vi "ChaseBoat.vi"(3 "Base Station data rec'd":string, 4 "inPriors":T1(array[cluster]), 5 "Tug letter":string="G") -> (0 "outPriors":T1(array[cluster]), 1 "predictedY":dbl, 2 "predictedX":dbl)   [LabVIEW 2012]
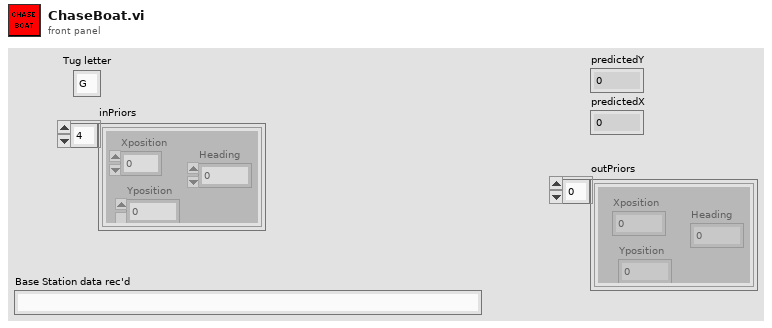
[diagram p1: front panel]
types:
  T1 = cluster{"Xposition":dbl, "Yposition":dbl, "Heading":dbl}[]
  T2 = cluster{"regular expression":string, i32, i32, i32}
  T3 = cluster{"Xposition":dbl, "Yposition":dbl, "Heading":dbl}
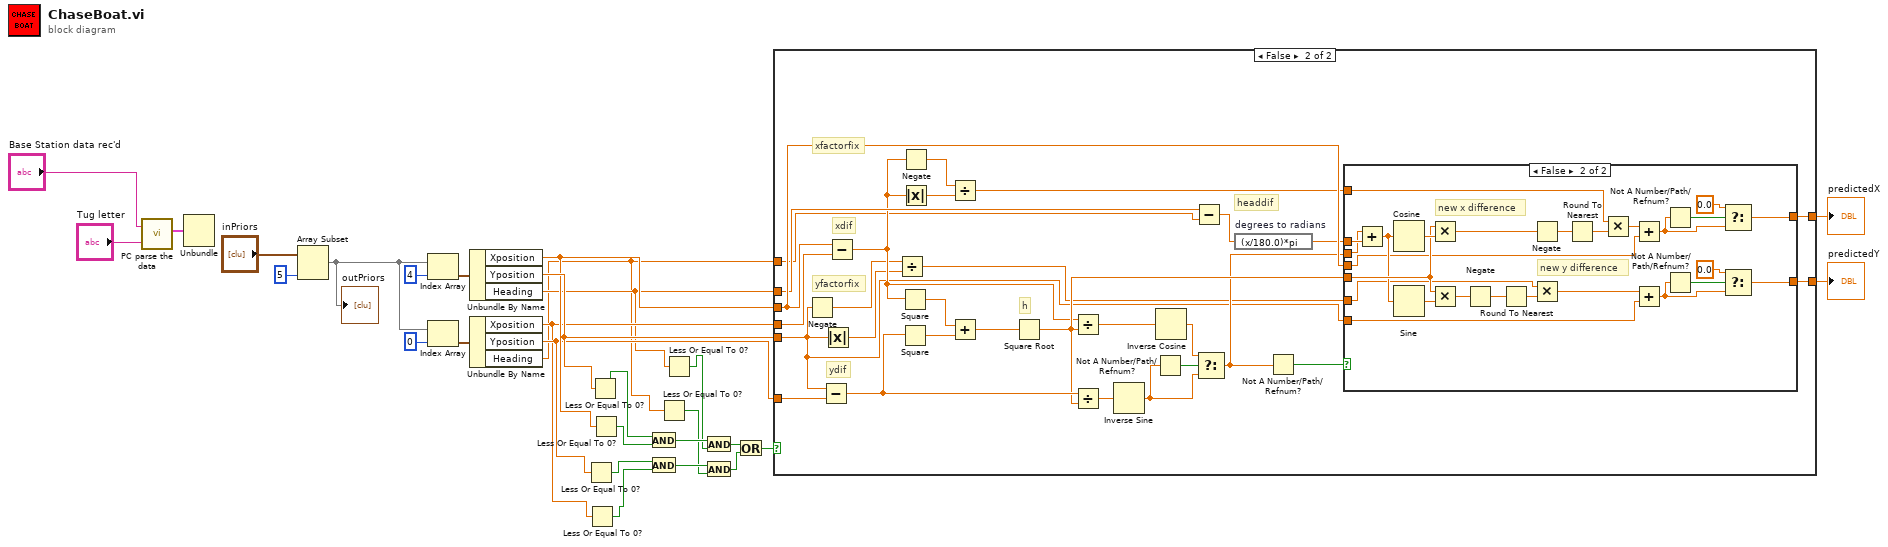
[diagram p0: block diagram]
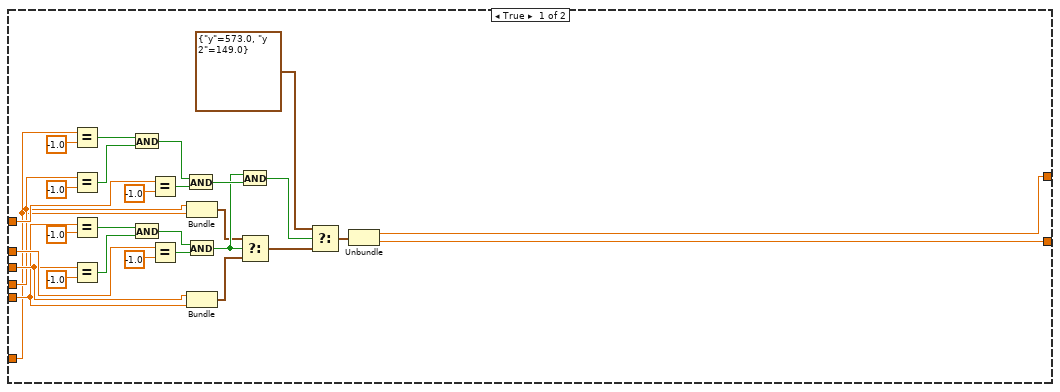
[diagram p2: hidden frame]
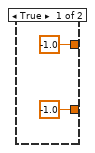
[diagram p3: hidden frame]
diagram:
  n1 = call "PC parse the data.vi"("Nav String"="Base Station data rec'd", "Tug"="Tug letter") -> ("Tug Location"=w27:T2)  [unwired: 3 out]
  n2 = Unbundle(w27) -> ()  [unwired: 4 out]
  n3 = Array Subset(array="inPriors", length=5) -> (w25:T1)  [unwired: 1 in]
  "outPriors" <- w25
  n4 = Index Array(array=w25, index=4) -> (element=w21:T3)
  n5 = Index Array(array=w25, index=0) -> (element=w22:T3)
  n6 = Unbundle By Name(w21) -> ("Xposition"=w9:dbl, "Yposition"=w12:dbl, "Heading"=w3:dbl)
  n7 = Unbundle By Name(w22) -> ("Xposition"=w5:dbl, "Yposition"=w7:dbl, "Heading"=w2:dbl)
  n8 = Less Or Equal To 0?(x=w7) -> (x <= 0?=w8:bool)
  n9 = Less Or Equal To 0?(x=w5) -> (x <= 0?=w6:bool)
  n10 = Less Or Equal To 0?(x=w12) -> (x <= 0?=w11:bool)
  n11 = Less Or Equal To 0?(x=w9) -> (x <= 0?=w10:bool)
  n12 = And(x=w11, y=w10) -> (x .and. y?=w17:bool)
  n13 = And(x=w8, y=w6) -> (x .and. y?=w16:bool)
  n14 = Less Or Equal To 0?(x=w2) -> (x <= 0?=w1:bool)
  n15 = Less Or Equal To 0?(x=w3) -> (x <= 0?=w4:bool)
  n16 = And(x=w17, y=w4) -> (x .and. y?=w14:bool)
  n17 = And(x=w16, y=w1) -> (x .and. y?=w15:bool)
  n18 = Or(x=w14, y=w15) -> (x .or. y?=w13:bool)
  n19 = case shown="False" w13 {
    tunnel: w5 -> [w36 w88]
    tunnel: w7 -> [w35 w87]
    tunnel: w9 -> [w39 w83]
    tunnel: [w30 w82] -> w19
    tunnel: [w31 w81] -> w18
    tunnel: w3 -> [w52 w70]
    tunnel: w12 -> [w38 w63]
    tunnel: w2 -> [w44 w60]
    frame True {
      n20 = Equal?(x=w35, y=-1.0) -> (x = y?=w50:bool)
      n21 = Equal?(x=w36, y=-1.0) -> (x = y?=w51:bool)
      n22 = Equal?(x=w38, y=-1.0) -> (x = y?=w58:bool)
      n23 = Equal?(x=w39, y=-1.0) -> (x = y?=w59:bool)
      n24 = And(x=w50, y=w51) -> (x .and. y?=w49:bool)
      n25 = And(x=w58, y=w59) -> (x .and. y?=w57:bool)
      n26 = Equal?(x=w44, y=-1.0) -> (x = y?=w48:bool)
      n27 = Equal?(x=w52, y=-1.0) -> (x = y?=w56:bool)
      n28 = And(x=w49, y=w48) -> (x .and. y?=w43:bool)
      n29 = Bundle("Xposition"=w36, "Yposition"=w35) -> (w34:cluster{"Xposition":dbl, "Yposition":dbl})  [unwired: 1 in]
      n30 = And(x=w57, y=w56) -> (x .and. y?=w40:bool)
      n31 = Bundle("Xposition"=w39, "Yposition"=w38) -> (w37:cluster{"Xposition":dbl, "Yposition":dbl})  [unwired: 1 in]
      n32 = And(x=w40, y=w43) -> (x .and. y?=w42:bool)
      n33 = Select(t=w34, s=w40, f=w37) -> (s? t:f=w33:cluster{"Xposition":dbl, "Yposition":dbl})
      n34 = Select(t=cluster{"y":dbl, "y 2":dbl} {"y"=573.0, "y 2"=149.0}, s=w42, f=w33) -> (s? t:f=w32:cluster{"Xposition":dbl, "Yposition":dbl})
      n35 = Unbundle(w32) -> ("Xposition"=w31:dbl, "Yposition"=w30:dbl)
    }
    frame False {
      # "yfactorfix"
      # "xfactorfix"
      # "h"
      # "xdif"
      # "ydif"
      # "headdif"
      n36 = Negate(x=w63) -> (-x=w65:dbl)
      n37 = Subtract(x=w63, y=w87) -> (x-y=w79:dbl)
      n38 = Absolute Value(x=w63) -> (abs(x)=w64:dbl)
      n39 = Subtract(x=w83, y=w88) -> (x-y=w68:dbl)
      n40 = Divide(x=w65, y=w64) -> (x/y=w62:dbl)
      n41 = Square(x=w68) -> (x^2=w86:dbl)
      n42 = Square(x=w79) -> (x^2=w85:dbl)
      n43 = Negate(x=w68) -> (-x=w67:dbl)
      n44 = Absolute Value(x=w68) -> (abs(x)=w66:dbl)
      n45 = Divide(x=w67, y=w66) -> (x/y=w61:dbl)
      n46 = Add(x=w86, y=w85) -> (x+y=w84:dbl)
      n47 = Square Root(x=w84) -> (sqrt(x)=w78:dbl)
      n48 = Divide(x=w68, y=w78) -> (x/y=w80:dbl)
      n49 = Divide(x=w79, y=w78) -> (x/y=w77:dbl)
      n50 = Inverse Sine(1:w77) -> (0:w75:dbl)
      n51 = Not A Number/Path/Refnum?(number/path/refnum=w75) -> (NaN/Path/Refnum?=w76:bool)
      n52 = Inverse Cosine(1:w80) -> (0:w74:dbl)
      n53 = Subtract(x=w70, y=w60) -> (x-y=w69:dbl)
      n54 = Select(t=w74, s=w76, f=w75) -> (s? t:f=w71:dbl)
      n55 = expression code="(x/180.0)*pi" "degrees to radians"(w69) -> (w73:dbl)
      n56 = Not A Number/Path/Refnum?(number/path/refnum=w71) -> (NaN/Path/Refnum?=w72:bool)
      n57 = case shown="False" w72 {
        tunnel: w83 -> [_ w107]
        tunnel: [-1.0 w98] -> w82
        tunnel: w63 -> [_ w108]
        tunnel: [-1.0 w95] -> w81
        tunnel: w78 -> [_ w112]
        tunnel: w73 -> [_ w111]
        tunnel: w71 -> [_ w110]
        tunnel: w62 -> [_ w93]
        tunnel: w61 -> [_ w104]
        frame True {
        }
        frame False {
          # "new x difference"
          # "new y difference"
          n58 = Add(x=w110, y=w111) -> (x+y=w109:dbl)
          n59 = Cosine(x=w109) -> (cos(x)=w115:dbl)
          n60 = Sine(x=w109) -> (sin(x)=w116:dbl)
          n61 = Multiply(x=w112, y=w115) -> (x*y=w92:dbl)
          n62 = Multiply(x=w112, y=w116) -> (x*y=w114:dbl)
          n63 = Negate(x=w114) -> (-x=w113:dbl)
          n64 = Round To Nearest(number=w113) -> (nearest integer value=w106:dbl)
          n65 = Negate(x=w92) -> (-x=w91:dbl)
          n66 = Multiply(x=w93, y=w106) -> (x*y=w105:dbl)
          n67 = Round To Nearest(number=w91) -> (nearest integer value=w103:dbl)
          n68 = Multiply(x=w104, y=w103) -> (x*y=w102:dbl)
          n69 = Add(x=w102, y=w107) -> (x+y=w94:dbl)
          n70 = Add(x=w105, y=w108) -> (x+y=w99:dbl)
          n71 = Not A Number/Path/Refnum?(number/path/refnum=w94) -> (NaN/Path/Refnum?=w97:bool)
          n72 = Not A Number/Path/Refnum?(number/path/refnum=w99) -> (NaN/Path/Refnum?=w101:bool)
          n73 = Select(t=0.0, s=w97, f=w94) -> (s? t:f=w95:dbl)
          n74 = Select(t=0.0, s=w101, f=w99) -> (s? t:f=w98:dbl)
        }
      }
    }
  }
  "predictedY" <- w19
  "predictedX" <- w18
